vi "getSnapperEvents.vi"(8 "error in (no error)":errorcluster, 11 "SnapperEvents in":refnum<class "SnapperEvents.lvclass">) -> (0 "error out":errorcluster, 2 "snapperEvents":T1, 3 "SnapperEvents out":refnum<class "SnapperEvents.lvclass">)   [LabVIEW 2011, in "Views.lvlib" / "Camera.lvlib" / "SnapperEvents.lvclass"]
uses:
  SnapperEvents.lvclass
  SnapperEvents.lvclass/SnapperEvents.ctl
  Camera.lvlib
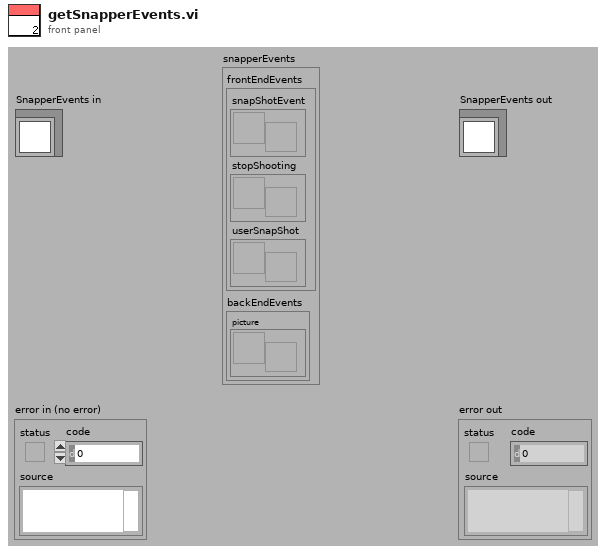
[diagram p1: front panel]
types:
  T1 = cluster{"frontEndEvents":cluster{"snapShotEvent":refnum<user-event>, "stopShooting":refnum<user-event>, "userSnapShot":refnum<user-event>}, "backEndEvents":cluster{"picture":refnum<user-event>}}
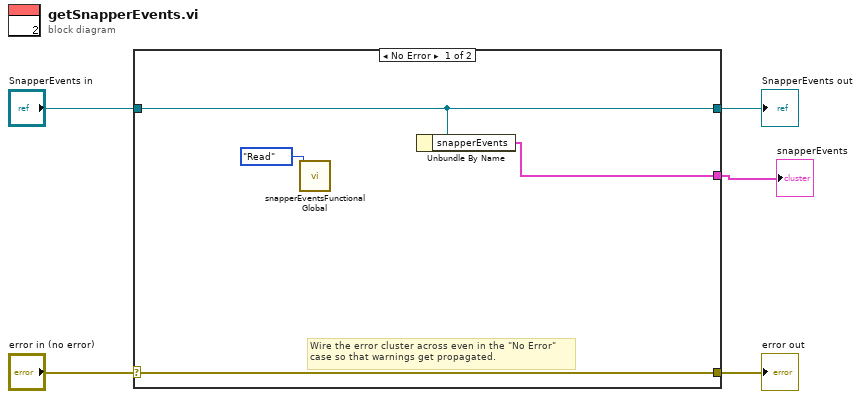
[diagram p0: block diagram]
diagram:
  n1 = case shown="No Error" "error in (no error)" {
    selector: "error in (no error)" -> [w9 w11]
    tunnel: [w9 w11] -> w4
    tunnel: [w7 w10] -> w2
    tunnel: "SnapperEvents in" -> [w7 w10]
    tunnel: [w6 _] -> w1
    frame No Error {
      # "Wire the error cluster across even in the \"No Error\"\ncase so that warnings get propagated."
      n2 = call "snapperEventsFunctionalGlobal.vi"("Action"=enum16{"Write", "Read"}."Read") -> ()  [unwired: 10 in, 1 out]
      n3 = Unbundle By Name(w7) -> ("snapperEvents"=w6:T1)
    }
    frame Error {
    }
  }
  "error out" <- w4
  "SnapperEvents out" <- w2
  "snapperEvents" <- w1
